vi "Cosine Window Coefficients.vi"(1 "window":T1(ring)) -> (0 "WinCoefficients":dbl[](array[numeric]) format="%0.2f")   [LabVIEW 2018, in "NI_AALPro.lvlib"]
uses:
  <vilib>/Analysis/NI_AALPro.lvlib
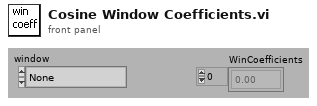
[diagram p1: front panel]
types:
  T1 = enum16{"None ", "Hanning", "Hamming", "Blackman-Harris", "Exact Blackman", "Blackman", "Flat Top", "4 Term B-Harris ", "7 Term B-Harris", "Low Sidelobe"}
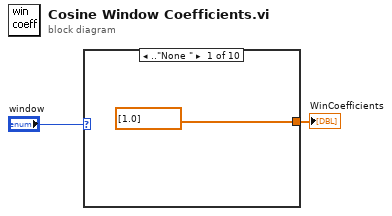
[diagram p0: block diagram]
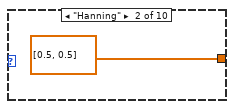
[diagram p2: hidden frame]
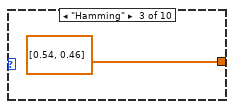
[diagram p3: hidden frame]
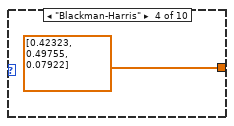
[diagram p4: hidden frame]
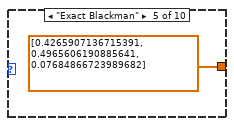
[diagram p5: hidden frame]
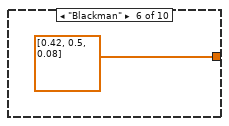
[diagram p6: hidden frame]
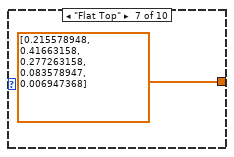
[diagram p7: hidden frame]
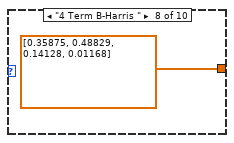
[diagram p8: hidden frame]
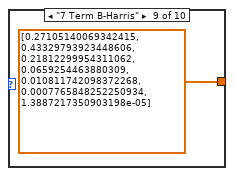
[diagram p9: hidden frame]
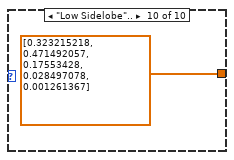
[diagram p10: hidden frame]
diagram:
  n1 = case shown="..\"None \"" "window" {
    tunnel: [dbl[] [1.0] ("Array") dbl[] [0.5, 0.5] ("Array") dbl[] [0.54, 0.46] ("Array") dbl[] [0.42323, 0.49755, 0.07922] ("Array") dbl[] [0.4265907136715391, 0.4965606190885641, 0.07684866723989682] ("Array") dbl[] [0.42, 0.5, 0.08] ("Array") dbl[] [0.215578948, 0.41663158, 0.277263158, 0.083578947, 0.006947368] ("Array") dbl[] [0.35875, 0.48829, 0.14128, 0.01168] ("Array") dbl[] [0.27105140069342415, 0.43329793923448606, 0.21812299954311062, 0.0659254463880309, 0.010811742098372268, 0.0007765848252250934, 1.3887217350903198e-05] ("Array") dbl[] [0.323215218, 0.471492057, 0.17553428, 0.028497078, 0.001261367] ("Output Array")] -> w1
    frame .."None " {
    }
    frame "Hanning" {
    }
    frame "Hamming" {
    }
    frame "Blackman-Harris" {
    }
    frame "Exact Blackman" {
    }
    frame "Blackman" {
    }
    frame "Flat Top" {
    }
    frame "4 Term B-Harris " {
    }
    frame "7 Term B-Harris" {
    }
    frame "Low Sidelobe".. {
    }
  }
  "WinCoefficients" <- w1
